vi "GEN_WriteError.vi"(6 "Error MSG":string="Error MSG", 7 "Name":string, 8 "error In":errorcluster, 9 "Success?":bool, 10 "Configuration Cluster In":T1={"General"={"Config.ini"=path "", "Default Logging Path"=path ""}, "Hardware"={"Global T VAR"="", "Global B VAR"="", "VISAS"={"GEN COM"="", "SCOPE COM"="", "VNA COM"=""}}, "Operation"={"Operation Mode"=enum."Idle-Off", "Status"="", "NewLog?"=FALSE, "OvenWarn"=FALSE, "Scope Settings"={"TimeBase"=0.0, "VerticalScale"=0.0}}}, 11 "Status Ref":refnum<vi>) -> (0 "error out":errorcluster, 2 "Config_Cluster Out":T1={"General"={"Config.ini"=path "", "Default Logging Path"=path ""}, "Hardware"={"Global T VAR"="", "Global B VAR"="", "VISAS"={"GEN COM"="", "SCOPE COM"="", "VNA COM"=""}}, "Operation"={"Operation Mode"=enum."Idle-Off", "Status"="", "NewLog?"=FALSE, "OvenWarn"=FALSE, "Scope Settings"={"TimeBase"=0.0, "VerticalScale"=4.0}}})   [LabVIEW 2021]
uses:
  Config_Cluster.ctl
  Mode_Enum.ctl
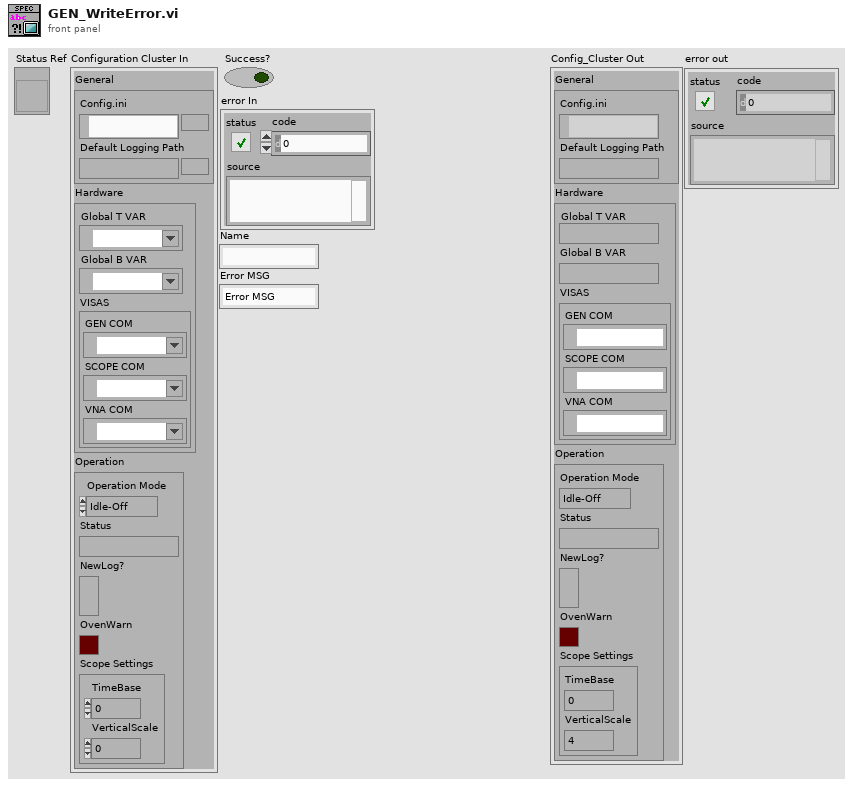
[diagram p1: front panel]
types:
  T1 = typedef "Config_Cluster.ctl" = cluster{"General":cluster{"Config.ini":path, "Default Logging Path":path}, "Hardware":cluster{"Global T VAR":refnum<k21>, "Global B VAR":refnum<k21>, "VISAS":cluster{"GEN COM":refnum<visa-resource-name>, "SCOPE COM":refnum<visa-resource-name>, "VNA COM":refnum<visa-resource-name>}}, "Operation":cluster{"Operation Mode":T2, "Status":string, "NewLog?":bool, "OvenWarn":bool, "Scope Settings":cluster{"TimeBase":dbl, "VerticalScale":dbl}}}
  T2 = typedef "Mode_Enum.ctl" = enum16{"OvenNRDY", "Logging", "Idle-Off", "Idle"}
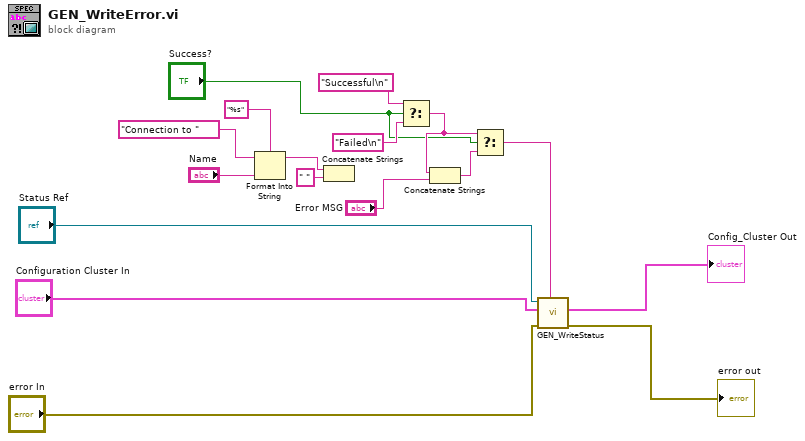
[diagram p0: block diagram]
diagram:
  n1 = Format Into String(format string="%s", initial string="Connection to ", "Name") -> (resulting string=w8:string)  [unwired: 1 in, 1 out]
  n2 = Concatenate Strings(w8, " " ("string")) -> ()  [unwired: 1 out]
  n3 = Select(t="Successful\n", s="Success?", f="Failed\n") -> (s? t:f=w11:string)
  n4 = Concatenate Strings(w11, "Error MSG") -> (w12:string)
  n5 = Select(t=w11, s="Success?", f=w12) -> (s? t:f=w9:string)
  n6 = call "GEN_WriteStatus.vi"("Input String"=w9, "error in (no error)"="error In", "Config_Cluster"="Configuration Cluster In", "Status Ref"="Status Ref") -> ("error out"=→"error out":errorcluster, "Config_Cluster Out"=→"Config_Cluster Out":T1)  [unwired: 6 in]
